vi "Disable Custom Device.vi"(8 "error in":errorcluster, 11 "custom device ref":T1 format="%.0x") -> (0 "error out":errorcluster, 3 "custom device ref out":T1 format="%.0x")   [LabVIEW 2020, in "AIM MIL-STD-1553 Scripting.lvlib"]
doc: "Disables the <b>custom device</b>, which ignores the compilation of the engine during deployment. \n\nThis is primarily used for troubleshooting purposes, to allow a user to stop custom device behavior without having to remove/recreate the custom device."
uses:
  AIM MIL-STD-1553 Scripting.lvlib
  <vilib>/NI VeriStand/Custom Device API/Custom Device Item Ref.ctl
  NationalInstruments.VeriStand.SystemDefinitionAPI
  Constants.vi
  <vilib>/NI VeriStand/Custom Device API/Custom Device API.lvlib
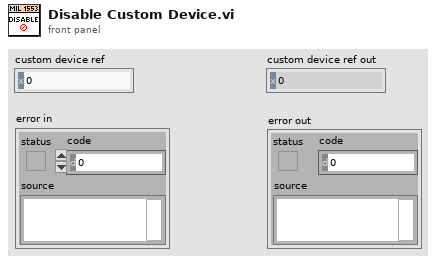
[diagram p1: front panel]
types:
  T1 = typedef "Custom Device API.lvlib/Custom Device Item Ref.ctl" = u64
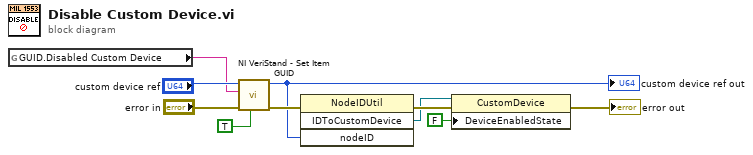
[diagram p0: block diagram]
diagram:
  n1 = global read "Constants.vi" "GUID.Disabled Custom Device"() -> (w1:string)
  n2 = call <vilib>:"NI VeriStand - Set Item GUID.vi"("Refresh System Explorer Tree? (F)"=TRUE, "error in (no error)"="error in", "GUID"=w1, "Item Ref in"="custom device ref") -> ("error out"=w9:errorcluster, "Item Ref out"=w3:T1)  [unwired: 6 in]
  "custom device ref out" <- w3
  n3 = invoke class="NodeIDUtil" method="IDToCustomDevice"(error in=w9, "nodeID"=w3) -> (error out=w8:errorcluster, "IDToCustomDevice"=w7:refnum<k24>)  [unwired: 2 in, 2 out]
  n4 = property class="CustomDevice"(reference=w7, error in=w8, "DeviceEnabledState"=FALSE) -> (error out=→"error out":errorcluster)  [unwired: 1 out]
